vi "Phasor Correct Complex Phasor (Single Calibration) v2.vi"(6 "Init? (T)":bool=TRUE, 8 "Error In":errorcluster, 10 "Calibration Phasor (m, phi, f, t0)":T1, 11 "Complex Phasor Array (V x H)":csg[][](array[numeric])) -> (0 "Error Out":errorcluster, 3 "Corrected Complex Phasor Array (V x H)":csg[][](array[numeric]), 4 "CPU (s)":dbl)   [LabVIEW 2021, in "Phasor.lvlib"]
uses:
  Phasor.lvlib
  Calibration Phasor (m, phi).ctl
  Time/Time.lvlib
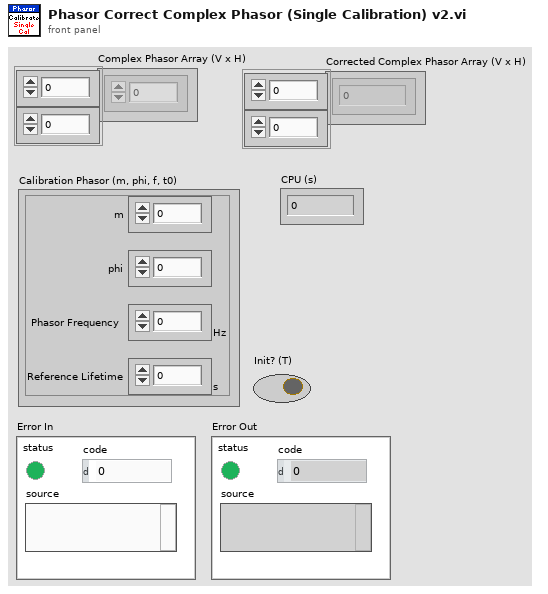
[diagram p1: front panel]
types:
  T1 = typedef "Phasor.lvlib/Calibration Phasor (m, phi).ctl" = cluster{"m":dbl, "phi":dbl, "Phasor Frequency":dbl[unit], "Reference Lifetime":dbl[unit]}
  T2 = cluster{"m":sgl, "phi":sgl, "Phasor Frequency":sgl[unit], "Reference Lifetime":sgl[unit]}
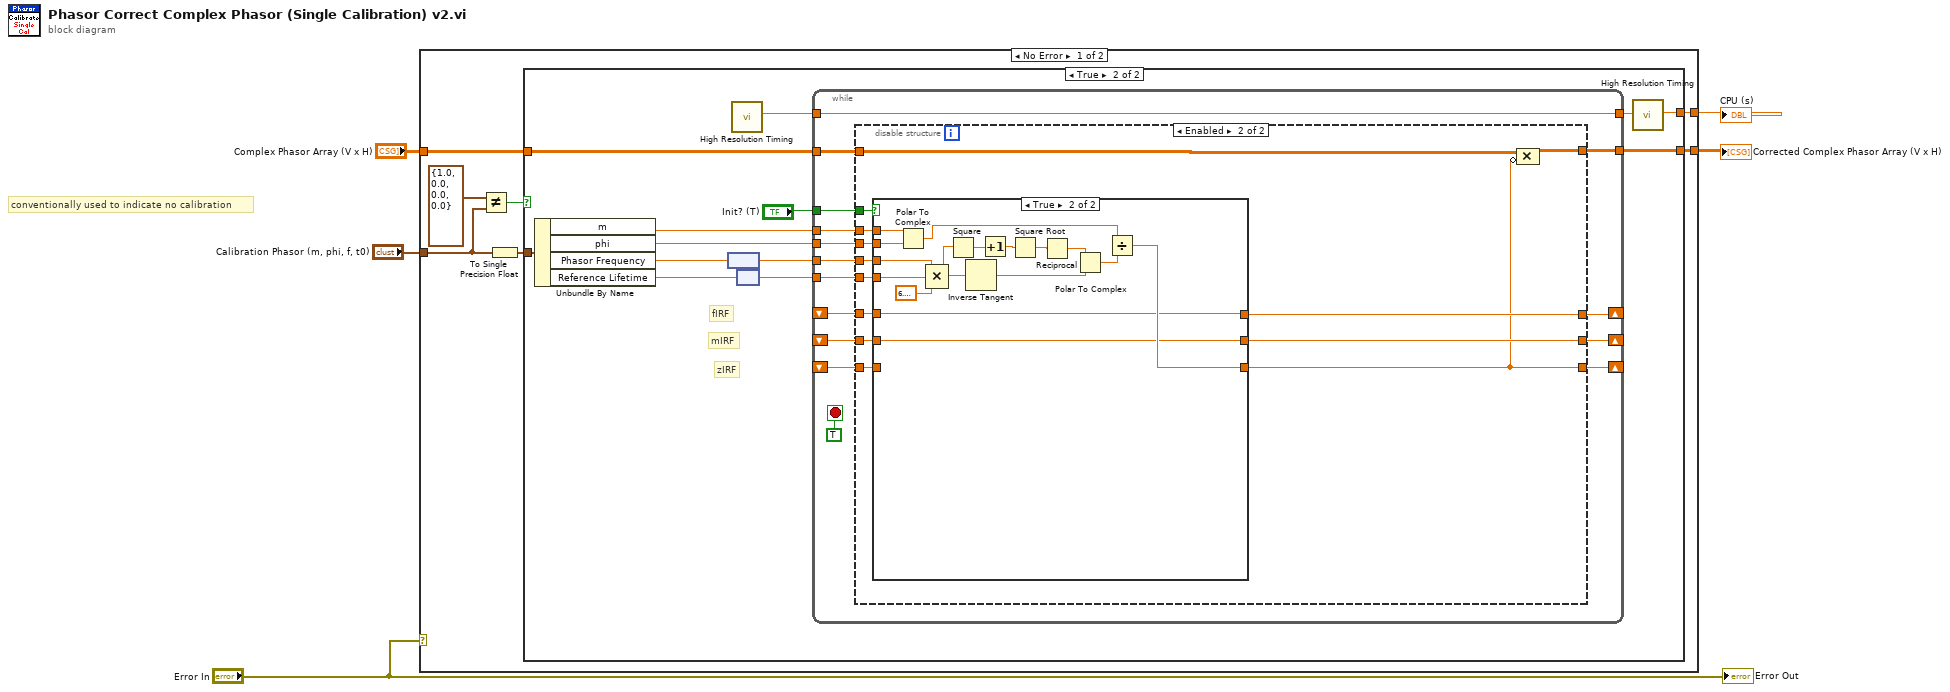
[diagram p0: block diagram]
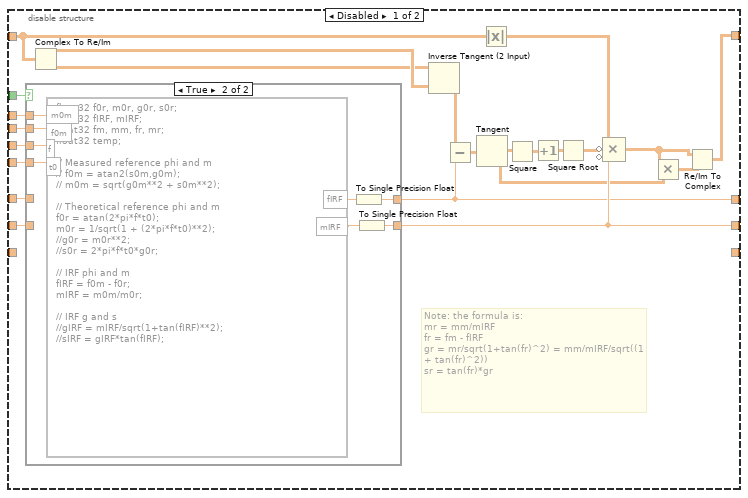
[diagram p3: hidden frame]
diagram:
  # "conventionally used to indicate no calibration"
  n1 = case shown="No Error" "Error In" {
    tunnel: "Complex Phasor Array (V x H)" -> [w12 w106]
    tunnel: [w11 _] -> w4
    tunnel: [w10 w106] -> w3
    tunnel: "Calibration Phasor (m, phi, f, t0)" -> [w8 _]
    frame No Error {
      n2 = Not Equal?(x=T1 {"m"=1.0, "phi"=0.0, "Phasor Frequency"=0.0, "Reference Lifetime"=0.0} ("Reference Phasor"), y=w8) -> (x != y?=w7:bool)
      n3 = To Single Precision Float(number=w8) -> (single precision float=w6:T2)
      n4 = case shown="True" w7 {
        tunnel: w12 -> [w13 w19]
        tunnel: [_ w16] -> w11
        tunnel: [w13 w15] -> w10
        tunnel: w6 -> [_ w14]
        frame False {
        }
        frame True {
          # "zIRF"
          # "mIRF"
          # "fIRF"
          n5 = Unbundle By Name(w14) -> ("m"=w26:sgl, "phi"=w25:sgl, "Phasor Frequency"=w24:sgl[unit], "Reference Lifetime"=w22:sgl[unit])
          n6 = node(w24) -> (w23:sgl)
          n7 = call "High Resolution Timing.vi"() -> ("elapsed (relative) seconds"=w18:dbl)  [unwired: 17 in, 2 out]
          n8 = node(w22) -> (w21:sgl)
          n9 = while {
            tunnel: "Init? (T)" -> [w40]
            tunnel: w26 -> [w39]
            tunnel: w25 -> [w38]
            tunnel: w23 -> [w37]
            tunnel: w21 -> [w36]
            shift-right: [w32] -> _
            shift-left: _ -> [w35]
            shift-right: [w33] -> _
            shift-left: _ -> [w34]
            tunnel: w18 -> [w31]
            tunnel: [w31] -> w17
            tunnel: w19 -> [w30]
            tunnel: [w29] -> w15
            shift-right: [w28] -> _
            shift-left: _ -> [w27]
            stop <- TRUE stop-if-true
            n10 = disable-structure shown="Enabled" {
              disable-tunnel: w40 -> [w63 w86]
              disable-tunnel: w39 -> [w62 w85]
              disable-tunnel: w38 -> [w61 w84]
              disable-tunnel: w37 -> [w60 w83]
              disable-tunnel: w36 -> [w59 w82]
              disable-tunnel: w35 -> [w58 w81]
              disable-tunnel: w34 -> [w57 w80]
              disable-tunnel: [w56 w79] -> w33
              disable-tunnel: [w54 w78] -> w32
              disable-tunnel: w30 -> [w47 w77]
              disable-tunnel: [w42 w76] -> w29
              disable-tunnel: [_ w74] -> w28
              disable-tunnel: w27 -> [_ w75]
              frame Disabled {
                # "Note: the formula is:\nmr = mm/mIRF\nfr = fm - fIRF\ngr = mr/sqrt(1+tan(fr)^2) = mm/mIRF/sqrt((1 + tan(fr)^2))\nsr = tan(fr)*gr"
                n11 = case shown="True" w63 {
                  tunnel: w62 -> [_ w73]
                  tunnel: w61 -> [_ w72]
                  tunnel: w60 -> [_ w71]
                  tunnel: w59 -> [_ w70]
                  tunnel: [w65 w67] -> w54
                  tunnel: [w64 w66] -> w56
                  tunnel: w58 -> [w65 _]
                  tunnel: w57 -> [w64 _]
                  frame False {
                  }
                  frame True {
                    n12 = formula code="float32 f0r, m0r, g0r, s0r;\nfloat32 fIRF, mIRF;\nfloat32 fm, mm, fr, mr;\nfloat32 temp;\n\n// Measured reference phi and m\n// f0m = atan2(s0m,g0m);\n// m0m = sqrt(g0m**2 + s0m**2);\n\n// Theoretical reference phi and m\nf0r = atan(2*pi*f*t0);\nm0r = 1/sqrt(1 + (2*pi*f*t0)**2);\n//g0r = m0r**2;\n//s0r = 2*pi*f*t0*g0r;\n\n// IRF phi and m\nfIRF = f0m - f0r;\nmIRF = m0m/m0r;\n\n// IRF g and s\n//gIRF = mIRF/sqrt(1+tan(fIRF)**2);\n//sIRF = gIRF*tan(fIRF);"("m0m"=w73, "f0m"=w72, "f"=w71, "t0"=w70) -> ("fIRF"=w69:sgl, "mIRF"=w68:sgl)
                    n13 = To Single Precision Float(number=w69) -> (single precision float=w67:sgl)
                    n14 = To Single Precision Float(number=w68) -> (single precision float=w66:sgl)
                  }
                }
                n15 = Complex To Re/Im(x + iy=w47) -> (x=w46:sgl[][], y=w45:sgl[][])
                n16 = Inverse Tangent (2 Input)(1:w46, 2:w45) -> (0:w55:sgl[][])
                n17 = Subtract(x=w55, y=w54) -> (x-y=w53:sgl[][])
                n18 = Tangent(1:w53) -> (0:w50:sgl[][])
                n19 = Absolute Value(x=w47) -> (abs(x)=w48:sgl[][])
                n20 = Square(x=w50) -> (x^2=w52:sgl[][])
                n21 = Increment(x=w52) -> (x+1=w51:sgl[][])
                n22 = Square Root(x=w51) -> (sqrt(x)=w49:sgl[][])
                n23 = Compound Arithmetic op=MULTIPLY(w48, invert w49, invert w56) -> (w44:sgl[][])
                n24 = Multiply(x=w44, y=w50) -> (x*y=w43:sgl[][])
                n25 = Re/Im To Complex(1:w43, 2:w44) -> (0:w42:csg[][])
              }
              frame Enabled {
                n26 = case shown="True" w86 {
                  tunnel: w85 -> [_ w96]
                  tunnel: w84 -> [_ w95]
                  tunnel: w83 -> [_ w105]
                  tunnel: w82 -> [_ w104]
                  tunnel: [w89 w90] -> w78
                  tunnel: [w88 w91] -> w79
                  tunnel: w81 -> [w89 w90]
                  tunnel: w80 -> [w88 w91]
                  tunnel: [w87 w92] -> w74
                  tunnel: w75 -> [w87 _]
                  frame False {
                  }
                  frame True {
                    n27 = Polar To Complex(1:w95, 2:w96) -> (0:w94:csg)
                    n28 = Compound Arithmetic op=MULTIPLY(w105, w104, sgl 6.2831855) -> (w102:sgl)
                    n29 = Square(x=w102) -> (x^2=w101:sgl)
                    n30 = Inverse Tangent(1:w102) -> (0:w98:sgl)
                    n31 = Increment(x=w101) -> (x+1=w100:sgl)
                    n32 = Square Root(x=w100) -> (sqrt(x)=w99:sgl)
                    n33 = Reciprocal(x=w99) -> (1/x=w97:sgl)
                    n34 = Polar To Complex(1:w98, 2:w97) -> (0:w93:csg)
                    n35 = Divide(x=w94, y=w93) -> (x/y=w92:csg)
                  }
                }
                n36 = Compound Arithmetic op=MULTIPLY(w77, invert w74) -> (w76:csg[][])
              }
            }
          }
          n37 = call "High Resolution Timing.vi"("relative seconds (NaN)"=w17) -> ("elapsed (relative) seconds"=w16:dbl)  [unwired: 16 in, 2 out]
        }
      }
    }
    frame Error {
    }
  }
  "Corrected Complex Phasor Array (V x H)" <- w3
  "CPU (s)" <- w4
  "Error Out" <- "Error In"
